vi "ClosestPoint.vi"(8 "Robot":cluster{"x":dbl, "y":dbl}, 11 "Path":cluster{"x":dbl, "y":dbl}[](array[cluster])) -> (2 "ClosestIndex":i32, 3 "Point":cluster{"x":dbl, "y":dbl})   [LabVIEW 2017]
doc: "Find the closest point to the robot"
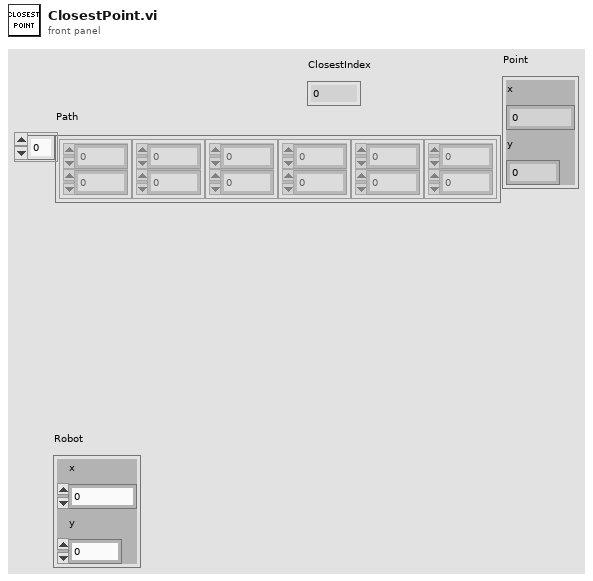
[diagram p1: front panel]
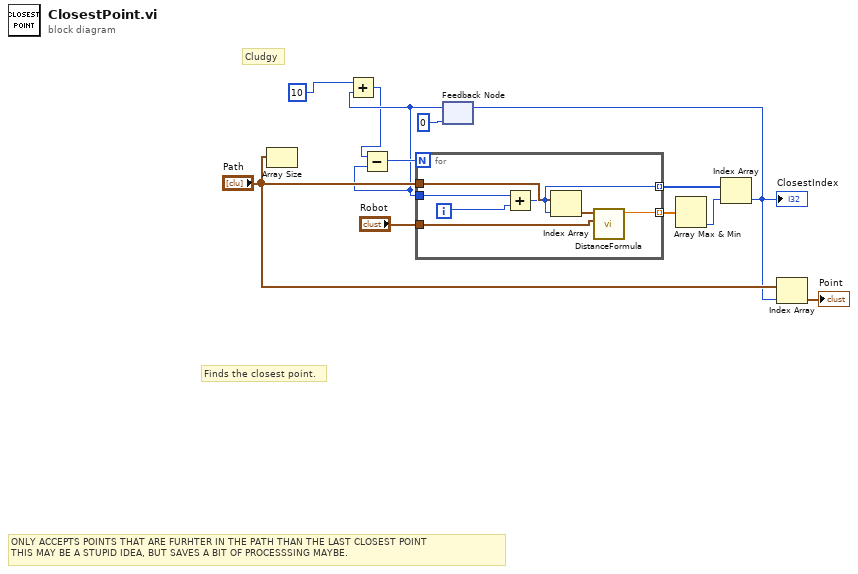
[diagram p0: block diagram]
diagram:
  # "Cludgy"
  # "ONLY ACCEPTS POINTS THAT ARE FURHTER IN THE PATH THAN THE LAST CLOSEST POINT\nTHIS MAY BE A STUPID IDEA, BUT SAVES A BIT OF PROCESSSING MAYBE."
  # "Finds the closest point."
  n1 = Array Size(array="Path") -> ()  [unwired: 1 out]
  n2 = feedback #1(0) -> (w2:i32)
  n3 = Add(x=10, y=w2) -> (x+y=w1:i32)
  n4 = Subtract(x=w1, y=w2) -> (x-y=w8:i32)
  n5 = for {
    N: w8 -> [_]
    tunnel: "Path" -> [w18]
    tunnel: "Robot" -> [w19]
    tunnel: w2 -> [w17]
    tunnel: [w15] -> w6 mode=indexing
    tunnel: [w14] -> w7 mode=indexing
    i -> [w13]
    n6 = Add(x=w17, y=w13) -> (x+y=w15:i32)
    n7 = Index Array(array=w18, index=w15) -> (element=w16:cluster{"x":dbl, "y":dbl})
    n8 = call "DistanceFormula.vi"("Point 2"=w19, "Point 1"=w16) -> ("Distance"=w14:dbl)  [unwired: 9 in]
  }
  n9 = Array Max & Min(array=w7) -> (min index (indices)=w5:i32)  [unwired: 3 out]
  n10 = Index Array(array=w6, index=w5) -> (element=w4:i32)
  "ClosestIndex" <- w4
  n11 = feedback-in #1(w4) -> ()
  n12 = Index Array(array="Path", index=w4) -> (element=→"Point":cluster{"x":dbl, "y":dbl})
